vi "Get Pin Status.vi"(8 "error in (no error)":errorcluster, 9 "Pin":dbl, 10 "Port":dbl, 11 "Cypress in":refnum<class "Cypress.lvclass">) -> (0 "error out":errorcluster, 3 "Cypress out":refnum<class "Cypress.lvclass">)   [LabVIEW 2020, in "Cypress.lvclass"]
uses:
  Cypress.lvclass
  7e1c2063-8ee1-4398-8073-dc09e10f7285.vi
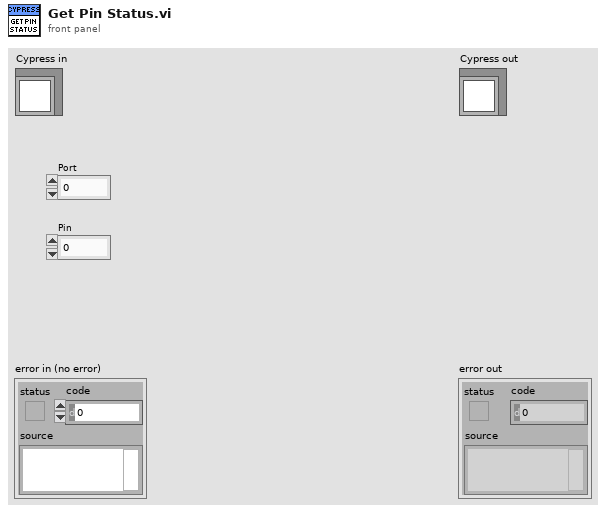
[diagram p1: front panel]
types:
  T1 = typedef "Serial device.lvclass/Brand combobox.ctl" = string
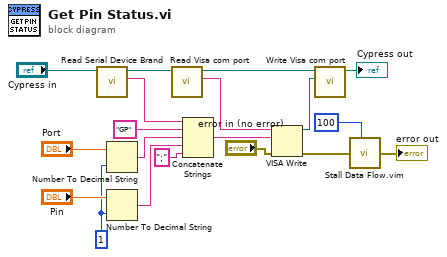
[diagram p0: block diagram]
diagram:
  w1 = i16 1 ("width (-)")
  n1 = call-dynamic "Read Serial Device Brand.vi"("Serial device in"="Cypress in") -> ("Serial Device Brand"=w3:T1, "Serial device out"=w17:refnum<class "Cypress.lvclass">)  [unwired: 8 in, 1 out]
  n2 = Number To Decimal String(number="Port", width (-)=w1) -> (decimal integer string=w15:string)
  n3 = Number To Decimal String(number="Pin", width (-)=w1) -> (decimal integer string=w13:string)
  n4 = call-dynamic "Read Visa com port.vi"("Serial device in"=w17) -> ("Visa com port"=w7:string, "Serial device out"=w18:refnum<class "Cypress.lvclass">)  [unwired: 8 in, 1 out]
  n5 = Concatenate Strings(w3, "GP" ("string"), w15, w13, ";" ("string")) -> (w2:string)
  n6 = VISA Write(VISA resource name=w7, write buffer=w2, error in (no error)="error in (no error)") -> (VISA resource name out=w6:refnum<visa-resource-name>, error out=w9:errorcluster)  [unwired: 1 out]
  n7 = call-dynamic "Write Visa com port.vi"("Visa com port"=w6, "Serial device in"=w18) -> ("Serial device out"=→"Cypress out":refnum<class "Cypress.lvclass">)  [unwired: 8 in, 1 out]
  n8 = call "Stall Data Flow.vim"("value in"=w9, "milliseconds to wait"=u32 100) -> ("value out"=→"error out":errorcluster)  [unwired: 1 out]
